vi "Exp06 Caracterizacao_Motor_exercicio.vi"() -> ()   [LabVIEW 2017]
doc: "This example demonstrates a simple PID position controller for a Quanser SRV-02 plant."
uses:
  <vilib>/Simulation/Scripting/Companion Diagram/SimConfigNode/SimParams.ctl
  <vilib>/Simulation/Scripting/Companion Diagram/SimConfigNode/_simSolvers.ctl
  <vilib>/Simulation/Implementation/Shared/SIMSCR Execution Mode.ctl
  <vilib>/Platform/TimedLoop/XDataNode/timing_clust.ctl
  <vilib>/Platform/TimedLoop/XDataNode/nitl_modes.ctl
  <vilib>/Platform/TimedLoop/XDataNode/wakeup.ctl
  <vilib>/Simulation/Param Hierarchy/Typedefs/SIMPH Param Control Actions.ctl
  <vilib>/Simulation/Implementation/Shared/NILVSim_ParamChanged.vi
  <vilib>/Simulation/Implementation/Shared/NILVSim_FinishedLate.vi
  <vilib>/Simulation/Implementation/Shared/NILVSIM_BeginStep.vi
  <vilib>/Simulation/Utility/Implementation/SIM Halt.vi
  <vilib>/Simulation/SignalArithmetic/Implementation/NILVSim Gain.llb/SIM Gain (scalar).vi
  <vilib>/Simulation/ContinuousLinear/Implementation/NILVSim Derivative.llb/SIM derivative (scalar).vi
  <vilib>/Simulation/DataSources/Implementation/NILVSim Step.llb/SIM Step (scalar).vi
  <vilib>/Simulation/DataSources/Implementation/NILVSim Signal Generator.llb/SIM Signal Generator (scalar).vi
  <vilib>/Simulation/ContinuousLinear/Implementation/NILVSim Transfer Function.llb/SIM Transfer Function Distributor (SISO).vi
  <vilib>/Simulation/ContinuousLinear/Implementation/NILVSim Transfer Function.llb/SIM Transfer Function Collector (SISO).vi
  <vilib>/Simulation/Utility/Implementation/NILVSim Collector.llb/SIM Collector (scalar).vi
  <vilib>/Simulation/Implementation/Shared/NILVSim_Manager.vi
  <vilib>/Utility/error.llb/Clear Errors.vi
  <vilib>/Simulation/Implementation/Shared/NILVSim_FinalizeModel.vi
  <vilib>/Simulation/Utility/Implementation/NILVSim Collector.llb/NILVSim Collector core (scalar).vi
  <vilib>/Simulation/Implementation/Shared/SIM Unbundle Sim Info.vi
  <vilib>/Simulation/Implementation/Shared/SIMSH Read Queue.vi
  <vilib>/Simulation/Implementation/Shared/NILVSim_Initialize.vi
  <vilib>/Simulation/Utility/Implementation/NILVSim Get Time and IsAcceptedStep.vi
  <vilib>/Simulation/Implementation/Shared/NILVSim_GetModelError.vi
  <vilib>/Simulation/Implementation/Shared/SIM Bundle Sim Info.vi
  <vilib>/Simulation/Scripting/Companion Diagram/SimConfigNode/SimDog.xnode
  <vilib>/Quanser/Rapid Control Prototyping Toolkit/hardware/HIL Immediate IO/_TypeSpecific/CL HIL Read Encoder (Scalar).vi
  <vilib>/Quanser/Rapid Control Prototyping Toolkit/hardware/HIL Immediate IO/CL HIL Read.vi
  <vilib>/Quanser/Rapid Control Prototyping Toolkit/hardware/HIL Immediate IO/_TypeSpecific/CL HIL Write Analog (Scalar).vi
  <vilib>/Quanser/Rapid Control Prototyping Toolkit/hardware/HIL Immediate IO/CL HIL Write.vi
  <vilib>/Platform/TimedLoop/XDataNode/XDataNode.xnode
  <vilib>/Simulation/Implementation/XNodeFramework/SimXNode/SimX.xnode
  <vilib>/Simulation/ContinuousLinear/Implementation/NILVSim Transfer Function.llb/SIM Transfer Function (SISO).vi
  <vilib>/Platform/TimedLoop/XDataNode/XDNodeRunTimeDep.lvlib
  <vilib>/Simulation/Implementation/Shared/NI_SIM_Implementation.lvlib
panel:
  out "XY Graph":cluster{"Time":dbl[], "Signal":dbl[]}[](graph)
  out "Degrau":dbl(graph)
  out "Velô":dbl(graph)
  out "Rads":i32
  out "Voltas":i32
  in  "Halt?":bool
  out "Error":errorcluster
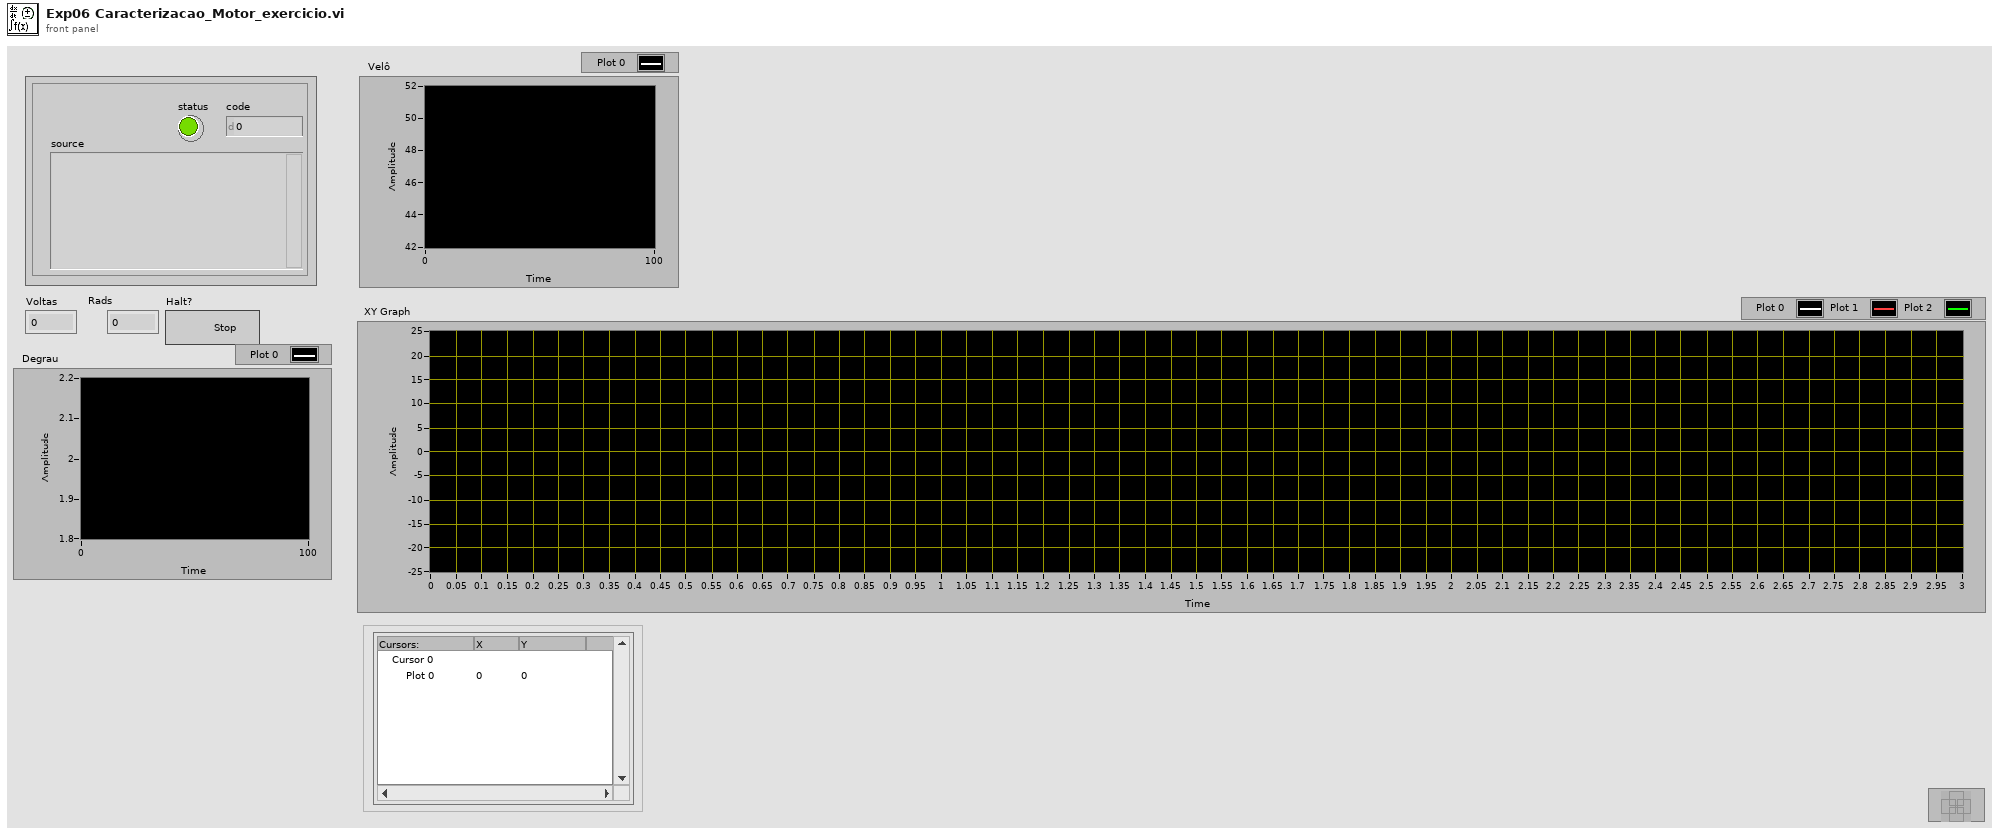
[diagram p1: front panel]
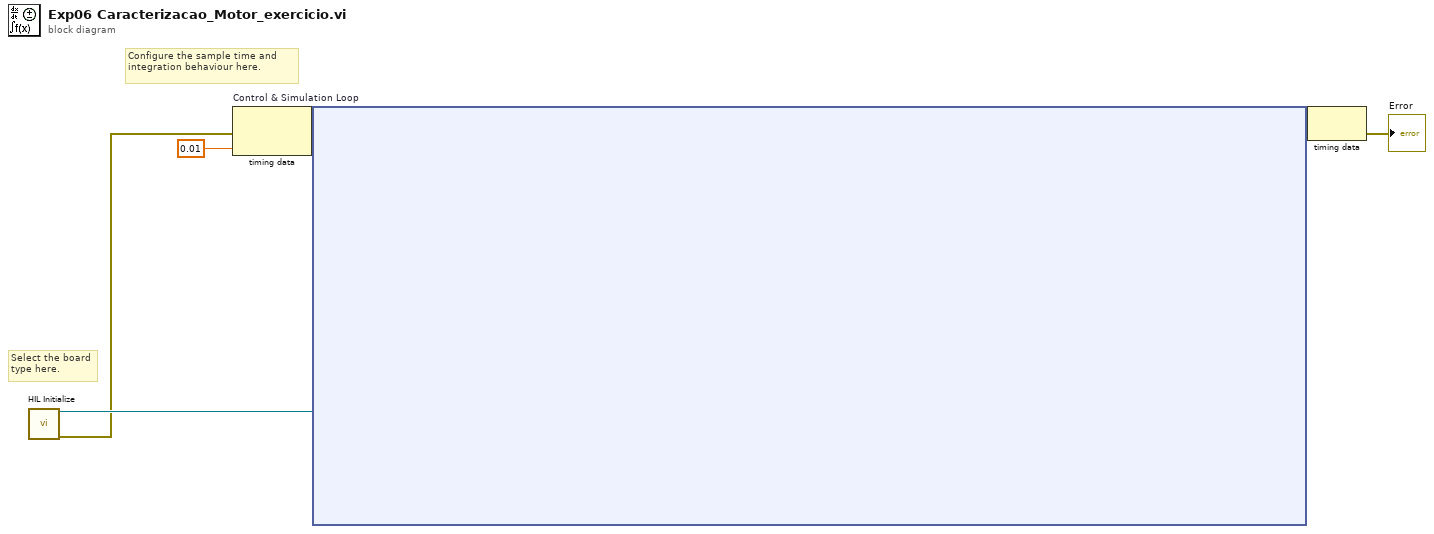
[diagram p0: block diagram]
diagram:
  # "Configure the sample time and integration behaviour here."
  # "Select the board\ntype here."
  n1 = call "HIL Initialize"() -> ("board out"=w4:refnum<class "HIL Board.lvclass">, "error out"=w1:errorcluster)  [unwired: 14 in]
  n2 = node-c288(w1, 0.01 ("Step Size (s)")) -> (w6:variant)
  n3 = node-c254 "Control & Simulation Loop"(w6, w4) -> (w5:variant)
  n4 = node-c288(w5) -> (→"Error":errorcluster)
